vi "Set ForeColor.vi"(8 "error in (no error)":errorcluster, 10 "Color.lvclass":refnum<class "Color.lvclass">, 11 "View in":refnum<class "ColumnHeader View.lvclass">) -> (0 "error out":errorcluster, 3 "View out":refnum<class "ColumnHeader View.lvclass">)   [LabVIEW 2024]
uses:
  ColumnHeader View.lvclass/ColumnHeader View.ctl
  Color/Color.lvclass
  ColumnHeader View.lvclass
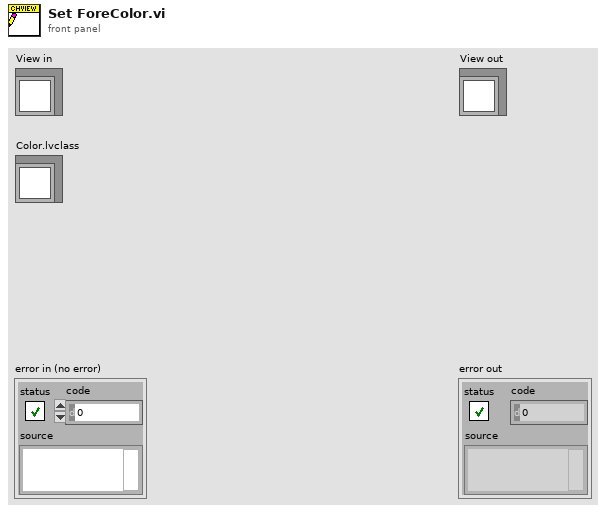
[diagram p1: front panel]
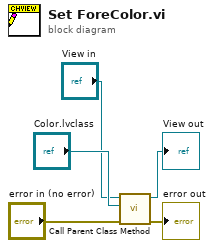
[diagram p0: block diagram]
diagram:
  n1 = call-parent "Call Parent Class Method"("error in (no error)"="error in (no error)", "Color.lvclass"="Color.lvclass", "View in"="View in") -> ("error out"=→"error out":errorcluster, "View out"=→"View out":refnum<class "ColumnHeader View.lvclass">)  [unwired: 7 in]
